vi "I2C_Send_Byte_Array_DAQ.vi"(1 "Tx.Byte.Count":i32, 2 "Tx.Array":u8[](array[numeric]) format="%02x") -> (0 "ALL.ACKS.OK":bool)   [LabVIEW 2022 SP3]
doc: "Petrus Prins 7 June 2026"
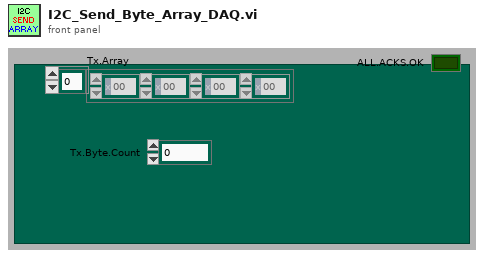
[diagram p1: front panel]
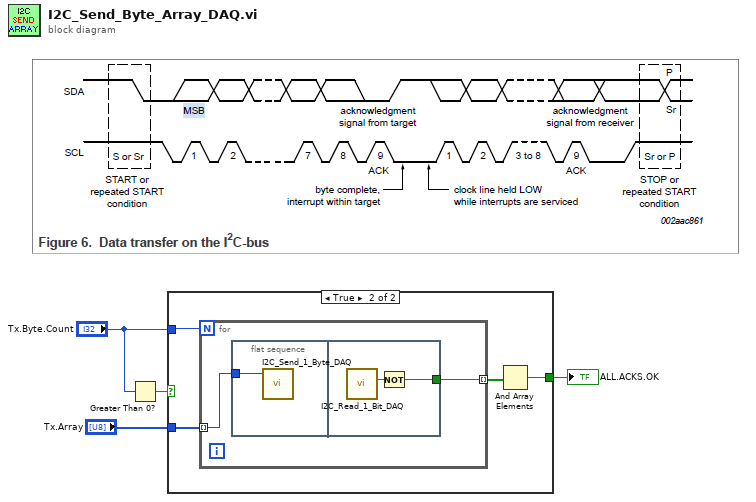
[diagram p0: block diagram]
diagram:
  n1 = Greater Than 0?(x="Tx.Byte.Count") -> (x > 0?=w4:bool)
  n2 = case shown="True" w4 {
    selector: w4 -> [w5 _]
    tunnel: "Tx.Byte.Count" -> [_ w9]
    tunnel: [w5 w7] -> w2
    tunnel: "Tx.Array" -> [_ w6]
    frame False {
    }
    frame True {
      n3 = for {
        N: w9 -> [_]
        tunnel: w6 -> [w11] mode=indexing
        tunnel: [w10] -> w8 mode=indexing
        n4 = flat-sequence {
          tunnel: w11 -> [w12]
          tunnel: [w13] -> w10
          frame #0 {
            n5 = call "I2C_Send_1_Byte_DAQ.vi"("Byte_To_Send"=w12) -> ()  [unwired: 2 in]
          }
          frame #1 {
            n6 = call "I2C_Read_1_Bit_DAQ.vi"() -> ("RX_Bit_Out"=w14:bool)  [unwired: 2 in]
            n7 = Not(x=w14) -> (.not. x?=w13:bool)
          }
        }
      }
      n8 = And Array Elements(Boolean array=w8) -> (logical AND=w7:bool)
    }
  }
  "ALL.ACKS.OK" <- w2
